vi "drive_straight_encoder.vi"(10 "Speed (ft/sec)":dbl, 11 "Distance":dbl) -> ()   [LabVIEW 2012]
uses:
  <vilib>/Rock Robotics/WPI/RobotDrive/WPI_RobotDriveMecanumDrive_Cartesian.vi
  <vilib>/Rock Robotics/WPI/RobotDrive/WPI_RobotDriveGetSetRefNum.vi
panel:
  # "Use Encoder to scale distance,"
  # "Speed setting +/- 1 Full Scale"
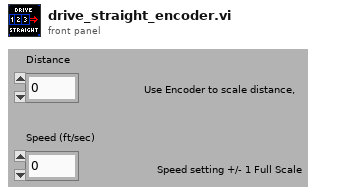
[diagram p1: front panel]
types:
  T1 = typedef "WPI_RobotDriveDevRef.ctl" = cluster{"DevStatus":errorcluster, "Motors[]":T2[], "Square Inputs":bool, "Max Output":dbl, "Isochronous":bool}
  T2 = typedef "WPI_MotorControlDeviceRef.ctl" = cluster{"DeviceStatus":errorcluster, "Type":enum16{"PWM", "CAN"}, "PWM":cluster{"Digital Module":T3, "PWM Channel":T4, "DeadBand":T5}, "CAN":cluster{"Device Number":u8, "Control Mode":T6, "Semaphore":T7, "Max Vout":dbl}, "Invert":bool, "TransformRef":T8, "InvTransformRef":T8}
  T3 = typedef "FPGA_TypedefDigitalModule.ctl" = enum16{"Digital Module 1", "Digital Module 2"}
  T4 = typedef "FPGA_DIOPWMChannel.ctl" = enum8{"PWM 1", "PWM 2", "PWM 3", "PWM 4", "PWM 5", "PWM 6", "PWM 7", "PWM 8", "PWM 9", "PWM 10", "Invalid"}
  T5 = typedef "WPI_PWMDeadband.ctl" = cluster{"Name":string, "maxPositivePwm":i32, "minPositivePwm":i32, "centerPwm":i32, "maxNegativePwm":i32, "minNegativePwm":i32, "angularRange":u16}
  T6 = typedef "WPI_CANJaguar_ControlMode.ctl" = enum8{"Percent VBus", "Current", "Speed", "Position", "Voltage"}
  T7 = typedef "Semaphore RefNum" = refnum<k1>
  T8 = typedef "WPI_PWMTransform_ConPane.ctl" = refnum<vi>
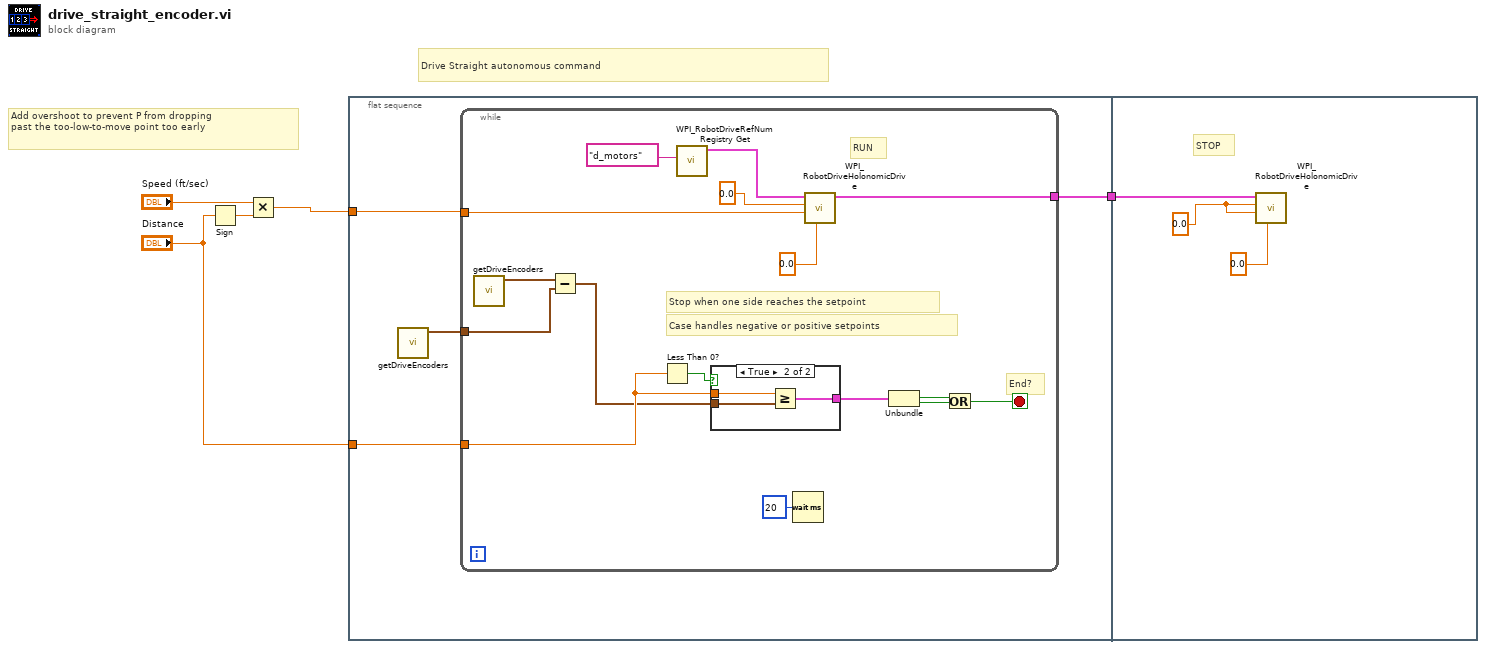
[diagram p0: block diagram]
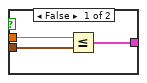
[diagram p2: hidden frame]
diagram:
  # "Drive Straight autonomous command"
  # "Add overshoot to prevent P from dropping\npast the too-low-to-move point too early"
  n1 = Sign(1:"Distance") -> (0:w3:dbl)
  n2 = Multiply(x="Speed (ft/sec)", y=w3) -> (x*y=w5:dbl)
  n3 = flat-sequence {
    tunnel: w5 -> [w8]
    tunnel: "Distance" -> [w7]
    tunnel: [w6] -> w1
    tunnel: w1 -> [w32]
    frame #0 {
      n4 = call "getDriveEncoders.vi"() -> ("Distance"=w9:cluster{"Left":dbl, "Right":dbl})  [unwired: 11 out]
      n5 = while {
        tunnel: w8 -> [w14]
        tunnel: w9 -> [w17]
        tunnel: w7 -> [w19]
        tunnel: [w10] -> w6
        stop <- w22 stop-if-true
        # "RUN"
        # "Case handles negative or positive setpoints"
        # "End?"
        # "Stop when one side reaches the setpoint"
        n6 = call "getDriveEncoders.vi"() -> ("Distance"=w18:cluster{"Left":dbl, "Right":dbl})  [unwired: 11 out]
        n7 = Subtract(x=w18, y=w17) -> (x-y=w16:cluster{"Left":dbl, "Right":dbl})
        n8 = Less Than 0?(x=w19) -> (x < 0?=w20:bool)
        n9 = call <vilib>:"WPI_RobotDriveRefNum Registry Get.vi"("refnum name"="d_motors") -> ("RobotDriveDevRef"=w13:T1)  [unwired: 1 in, 9 out]
        n10 = case shown="True" w20 {
          tunnel: w19 -> [w28 w31]
          tunnel: w16 -> [w27 w30]
          tunnel: [w26 w29] -> w25
          frame False {
            n11 = Less Or Equal?(x=w28, y=w27) -> (x <= y?=w26:cluster{"Left":bool, "Right":bool})
          }
          frame True {
            n12 = Greater Or Equal?(x=w31, y=w30) -> (x >= y?=w29:cluster{"Left":bool, "Right":bool})
          }
        }
        n13 = Wait (ms)(milliseconds to wait=u32 20) -> ()  [unwired: 1 out]
        n14 = call-poly <vilib>:"WPI_RobotDriveHolonomicDrive.vi"("Rotation"=0.0, "Y"=w14, "X"=0.0, "RobotDriveDevRef"=w13) -> ("RobotDriveDevRef"=w10:T1)  [unwired: 5 in, 2 out]
        n15 = Unbundle(w25) -> ("Left"=w24:bool, "Right"=w23:bool)
        n16 = Or(x=w24, y=w23) -> (x .or. y?=w22:bool)
      }
    }
    frame #1 {
      w33 = 0.0 ("X")
      # "STOP"
      n17 = call-poly <vilib>:"WPI_RobotDriveHolonomicDrive.vi"("Rotation"=0.0, "Y"=w33, "X"=w33, "RobotDriveDevRef"=w32) -> ()  [unwired: 5 in, 3 out]
    }
  }
